vi "CPU_MEM_read_mem_16.vi"(11 "registers":T1={"A"=0, "X"=0, "Y"=0, "SP"=253, "PC"=0, "P"=36} {"P" format="%08b"; "PC" format="%04x"; "SP" format="%02x"; "Y" format="%02x"; "X" format="%02x"; "A" format="%02x"}) -> (2 "value":u16 format="%04x", 3 "registers":T1={"A"=0, "X"=0, "Y"=0, "SP"=253, "PC"=0, "P"=36} {"P" format="%08b"; "PC" format="%04x"; "SP" format="%02x"; "Y" format="%02x"; "X" format="%02x"; "A" format="%02x"})   [LabVIEW 2018]
uses:
  CPU_registers.ctl
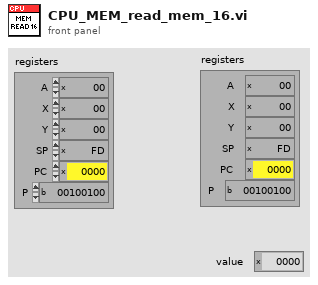
[diagram p1: front panel]
types:
  T1 = typedef "CPU_registers.ctl" = cluster{"A":u8, "X":u8, "Y":u8, "SP":u8, "PC":u16, "P":u8}
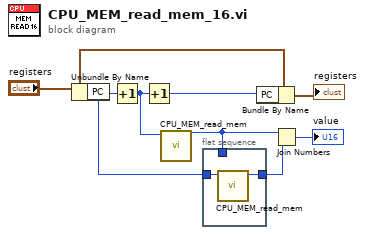
[diagram p0: block diagram]
diagram:
  n1 = Unbundle By Name("registers") -> ("PC"=w7:u16)
  n2 = Increment(x=w7) -> (x+1=w3:u16)
  n3 = Increment(x=w3) -> (x+1=w5:u16)
  n4 = call "CPU_MEM_read_mem.vi"("address"=w3) -> ("value out"=w1:u8)  [unwired: 10 in]
  n5 = flat-sequence {
    tunnel: w7 -> [w10]
    tunnel: [w9] -> w2
    tunnel: w1 -> [_]
    frame #0 {
      n6 = call "CPU_MEM_read_mem.vi"("address"=w10) -> ("value out"=w9:u8)  [unwired: 10 in]
    }
  }
  n7 = Bundle By Name(cluster="registers", "PC"=w5) -> (→"registers":T1)
  n8 = Join Numbers(hi=w1, lo=w2) -> ((hi.lo)=→"value":u16)
